vi "Periodic Tasks.vi"(8 "error in":errorcluster) -> ()   [LabVIEW 2017]
doc: "This VI runs in parallel to other robot code. It can contain as many user-defined periodic loops as you need. These can carry out PID or other sorts of timed response."
uses:
  <vilib>/Rock Robotics/WPI/Utilities/WPI_GetSetVariantRefNum.vi
  Robot Global Data.vi
  <vilib>/Rock Robotics/Network Tables/NT Write Number.vi
  <vilib>/Rock Robotics/Network Tables/NT Write Boolean.vi
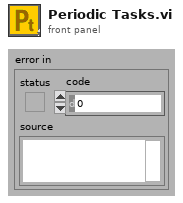
[diagram p1: front panel]
types:
  T1 = typedef "WPI_JoystickDevRef.ctl" = cluster{"Device":T2}
  T2 = typedef "WPI_JoystickDeviceEnum.ctl" = enum16{"USB 0", "USB 1", "USB 2", "USB 3", "USB 4", "USB 5"}
  T3 = typedef "WPI_GyroDevRef.ctl" = cluster{"DevStatus":errorcluster, "Analog Channel":T4, "Gain (VoltsPerDegree/Second)":dbl, "Gyro Type":enum16{"Analog", "XRS450"}, "Handle":i32, "SPI Bus":T5, "Device Found":bool, "Sample Rate":dbl, "Calibrate On Open":bool, "Offset":dbl}
  T4 = typedef "FPGA_AIChannel.ctl" = enum8{"AI 0", "AI 1", "AI 2", "AI 3", "AI MXP 0", "AI MXP 1", "AI MXP 2", "AI MXP 3", "Invalid"}
  T5 = typedef "spi_bus.ctl" = enum16{"SPI On-Board, CS0", "SPI On-Board, CS1", "SPI On-Board, CS2", "SPI On-Board, CS3", "SPI MXP", "Invalid"}
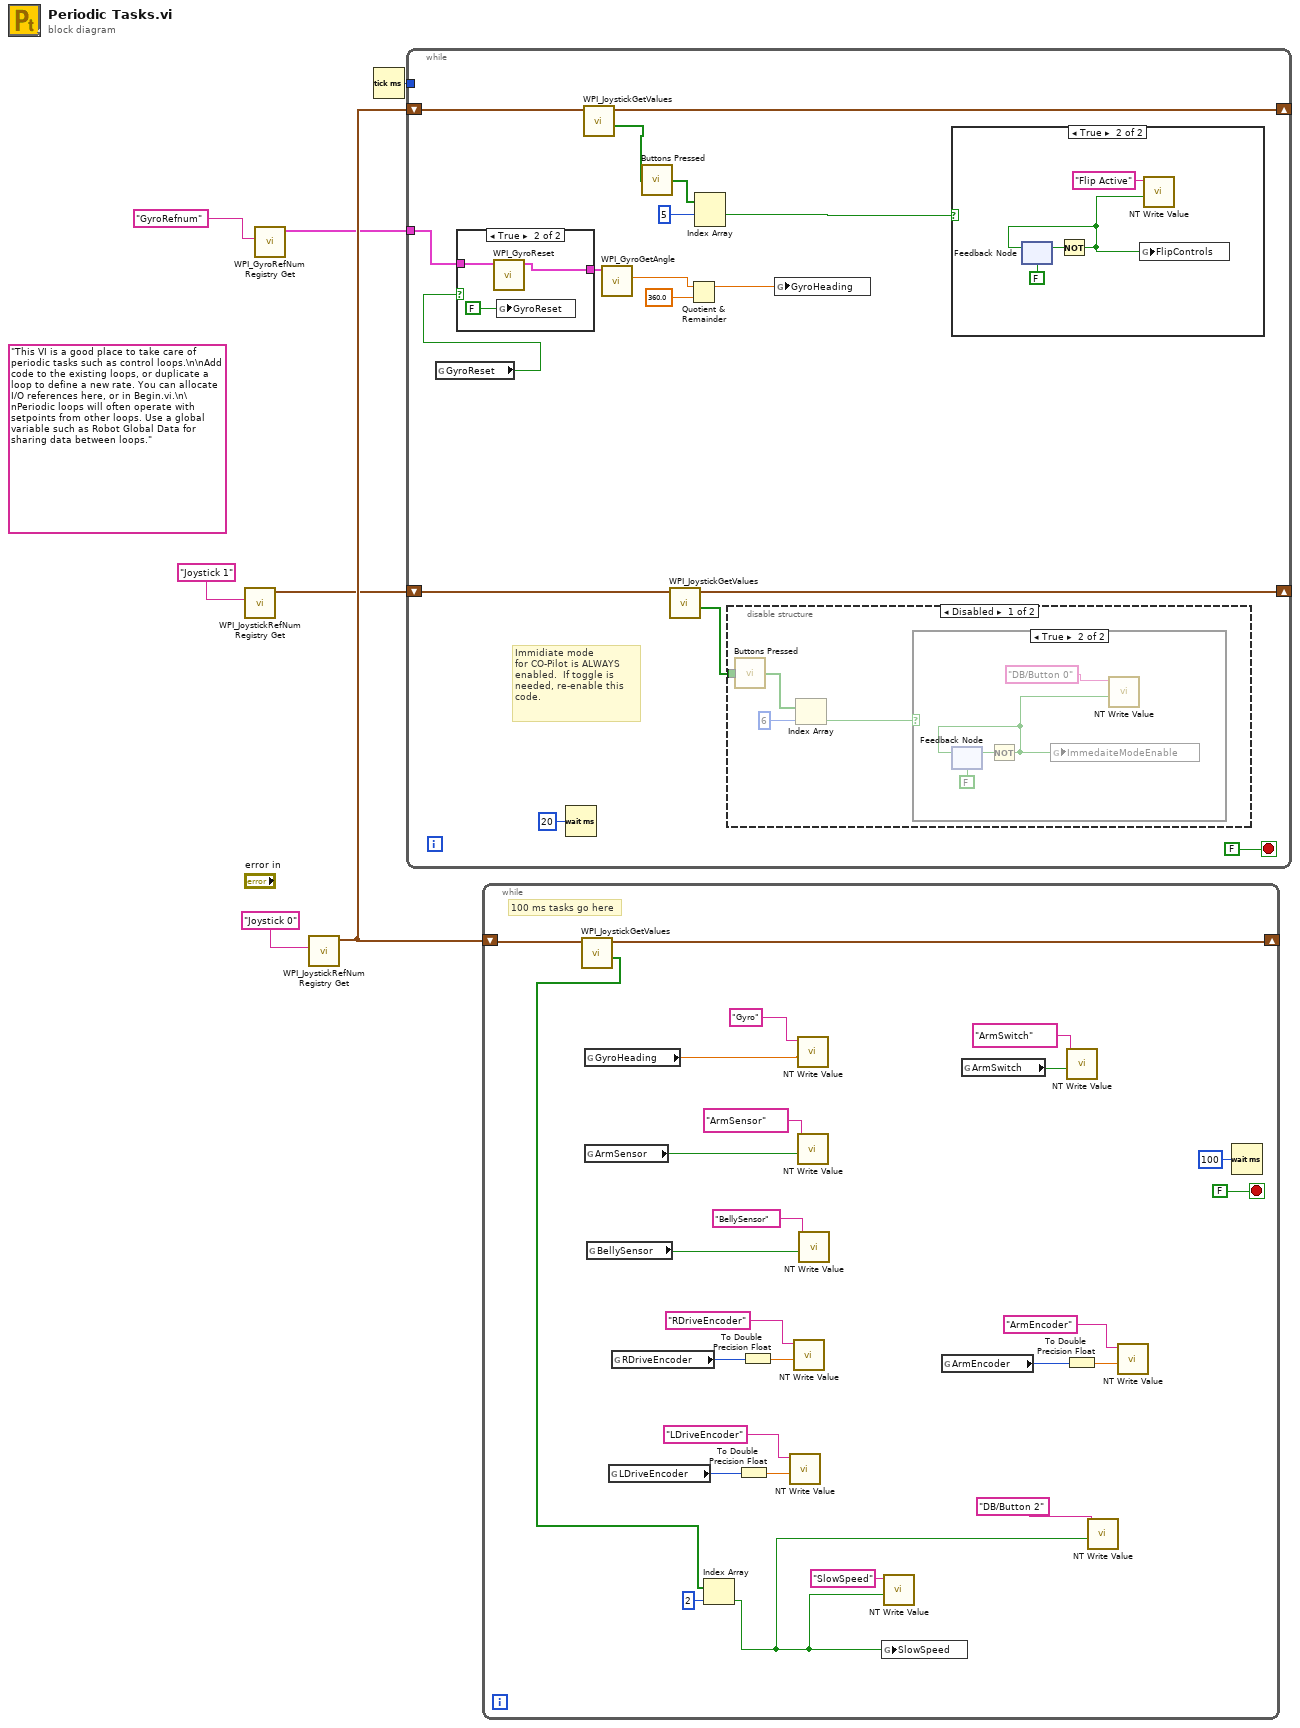
[diagram p0: block diagram]
diagram:
  (unwired) "This VI is a good place to take care of periodic tasks such as control loops.\n\nAdd code to the existing loops, or duplicate a loop to define a new rate. You can allocate I/O references here, or in Begin.vi.\n\nPeriodic loops will often operate with setpoints from other loops. Use a global variable such as Robot Global Data for sharing data between loops."
  n1 = call <vilib>:"WPI_JoystickRefNum Registry Get.vi"("refnum name"="Joystick 1") -> ("JoystickDevRef"=w1:T1)  [unwired: 1 in, 9 out]
  n2 = call <vilib>:"WPI_GyroRefNum Registry Get.vi"("refnum name"="GyroRefnum") -> ("GyroDevRef"=w3:T3)  [unwired: 9 in, 1 out]
  n3 = call <vilib>:"WPI_JoystickRefNum Registry Get.vi"("refnum name"="Joystick 0") -> ("JoystickDevRef"=w6:T1)  [unwired: 1 in, 9 out]
  n4 = Tick Count (ms)() -> (millisecond timer value=w5:u32)
  n5 = while {
    shift-right: [w19] -> _
    shift-left: w6 -> [w20]
    tunnel: w5 -> [_]
    tunnel: w3 -> [w12]
    shift-right: [w10] -> _
    shift-left: w1 -> [w11]
    stop <- FALSE stop-if-true
    # "Immidiate mode\nfor CO-Pilot is ALWAYS\nenabled.  If toggle is\nneeded, re-enable this\ncode."
    n6 = global read "Robot Global Data.vi" "GyroReset"() -> (w14:bool)
    n7 = case shown="True" w14 {
      tunnel: [w33 w35] -> w13
      tunnel: w12 -> [w33 w34]
      frame False {
      }
      frame True {
        n8 = call <vilib>:"WPI_GyroReset.vi"("GyroDevRef"=w34) -> ("GyroDevRef"=w35:T3)  [unwired: 9 in, 1 out]
        n9 = global write "Robot Global Data.vi" "GyroReset"(FALSE ("GyroReset")) -> ()
      }
    }
    n10 = Wait (ms)(milliseconds to wait=u32 20) -> ()  [unwired: 1 out]
    n11 = call <vilib>:"WPI_JoystickGetValues.vi"("JoystickDevRef"=w20) -> ("Buttons"=w8:bool[], "JoystickDevRef"=w19:T1)  [unwired: 6 in, 3 out]
    n12 = call <vilib>:"WPI_GyroGetAngle.vi"("GyroDevRef"=w13) -> ("Angle"=w16:dbl)  [unwired: 6 in, 4 out]
    n13 = call "Buttons Pressed.vi"("Button Values"=w8) -> ("Button Presses"=w21:bool[])
    n14 = call <vilib>:"WPI_JoystickGetValues.vi"("JoystickDevRef"=w11) -> ("Buttons"=w9:bool[], "JoystickDevRef"=w10:T1)  [unwired: 6 in, 3 out]
    n15 = Quotient & Remainder(x=w16, y=360.0) -> (x-y*floor(x/y)=w15:dbl)  [unwired: 1 out]
    n16 = Index Array(array=w21, index #1=5 ("index")) -> (element #1=w18:bool)  [unwired: 1 in, 1 out]
    n17 = disable-structure shown="Disabled" {
      disable-tunnel: w9 -> [w26 _]
      frame Disabled {
        n18 = call "Buttons Pressed.vi"("Button Values"=w26) -> ("Button Presses"=w28:bool[])
        n19 = Index Array(array=w28, index=6) -> (element=w25:bool)
        n20 = case shown="True" w25 {
          frame False {
          }
          frame True {
            n21 = feedback #1(FALSE) -> (w30:bool)
            n22 = Not(x=w30) -> (.not. x?=w29:bool)
            n23 = feedback-in #1(w29) -> ()
            n24 = global write "Robot Global Data.vi" "ImmedaiteModeEnable"(w29) -> ()
            n25 = call-poly <vilib>:"NT Write Value.vi"("Boolean"=w29, "Name"="DB/Button 0") -> ()  [unwired: 9 in, 1 out]
          }
        }
      }
      frame Enabled {
      }
    }
    n26 = global write "Robot Global Data.vi" "GyroHeading"(w15) -> ()
    n27 = case shown="True" w18 {
      frame False {
      }
      frame True {
        n28 = feedback #2(FALSE) -> (w38:bool)
        n29 = Not(x=w38) -> (.not. x?=w37:bool)
        n30 = feedback-in #2(w37) -> ()
        n31 = global write "Robot Global Data.vi" "FlipControls"(w37) -> ()
        n32 = call-poly <vilib>:"NT Write Value.vi"("Boolean"=w37, "Name"="Flip Active") -> ()  [unwired: 9 in, 1 out]
      }
    }
  }
  n33 = while {
    shift-right: [w63] -> _
    shift-left: w6 -> [w64]
    stop <- FALSE stop-if-true
    # "100 ms tasks go here"
    n34 = call <vilib>:"WPI_JoystickGetValues.vi"("JoystickDevRef"=w64) -> ("Buttons"=w43:bool[], "JoystickDevRef"=w63:T1)  [unwired: 6 in, 3 out]
    n35 = global read "Robot Global Data.vi" "GyroHeading"() -> (w62:dbl)
    n36 = global read "Robot Global Data.vi" "ArmSensor"() -> (w60:bool)
    n37 = global read "Robot Global Data.vi" "BellySensor"() -> (w57:bool)
    n38 = global read "Robot Global Data.vi" "LDriveEncoder"() -> (w47:i32)
    n39 = global read "Robot Global Data.vi" "RDriveEncoder"() -> (w55:i32)
    n40 = Index Array(array=w43, index=2) -> (element=w41:bool)
    n41 = To Double Precision Float(number=w47) -> (double precision float=w46:dbl)
    n42 = To Double Precision Float(number=w55) -> (double precision float=w54:dbl)
    n43 = call-poly <vilib>:"NT Write Value.vi"("Numeric"=w46, "Name"="LDriveEncoder") -> ()  [unwired: 9 in, 1 out]
    n44 = call-poly <vilib>:"NT Write Value.vi"("Numeric"=w54, "Name"="RDriveEncoder") -> ()  [unwired: 9 in, 1 out]
    n45 = call-poly <vilib>:"NT Write Value.vi"("Numeric"=w62, "Name"="Gyro") -> ()  [unwired: 9 in, 1 out]
    n46 = call-poly <vilib>:"NT Write Value.vi"("Boolean"=w60, "Name"="ArmSensor") -> ()  [unwired: 9 in, 1 out]
    n47 = call-poly <vilib>:"NT Write Value.vi"("Boolean"=w57, "Name"="BellySensor") -> ()  [unwired: 9 in, 1 out]
    n48 = global write "Robot Global Data.vi" "SlowSpeed"(w41) -> ()
    n49 = call-poly <vilib>:"NT Write Value.vi"("Boolean"=w41, "Name"="SlowSpeed") -> ()  [unwired: 9 in, 1 out]
    n50 = global read "Robot Global Data.vi" "ArmEncoder"() -> (w52:i32)
    n51 = global read "Robot Global Data.vi" "ArmSwitch"() -> (w50:bool)
    n52 = call-poly <vilib>:"NT Write Value.vi"("Boolean"=w50, "Name"="ArmSwitch") -> ()  [unwired: 9 in, 1 out]
    n53 = To Double Precision Float(number=w52) -> (double precision float=w51:dbl)
    n54 = call-poly <vilib>:"NT Write Value.vi"("Boolean"=w41, "Name"="DB/Button 2") -> ()  [unwired: 9 in, 1 out]
    n55 = call-poly <vilib>:"NT Write Value.vi"("Numeric"=w51, "Name"="ArmEncoder") -> ()  [unwired: 9 in, 1 out]
    n56 = Wait (ms)(milliseconds to wait=u32 100) -> ()  [unwired: 1 out]
  }
